vi "Icai 105v2.vi"() -> ()   [LabVIEW 2022 SP3]
uses:
  <vilib>/Utility/error.llb/DialogType.ctl
  <vilib>/DAQmx/write.llb/DAQmx Write (Analog DBL 1Chan 1Samp).vi
  <vilib>/DAQmx/write.llb/DAQmx Write (Analog Wfm 1Chan NSamp).vi
  <vilib>/DAQmx/create/channels.llb/DAQmx Create Channel (AO-Voltage-Basic).vi
  <vilib>/DAQmx/miscellaneous.llb/DAQmx Fill In Error Info.vi
  <vilib>/Waveform/WDTOps.llb/WDT Append Waveforms DBL.vi
  <vilib>/measure/NI_MABase.lvlib
panel:
  out "task out 2":refnum<k21> caption="task out"
  out "error out 2":errorcluster caption="error out (DAQ)"
  in  "Fs":dbl=1000000.0
  in  "?":T1(ring)=enum."Triangle Wave"
  in  "amplitude":dbl=1.0 format="%0.2p"
  in  "flat/ramp":bool
  in  "Ampl-RF \nend":dbl
  in  "Ampl-MW end":dbl=-1.0
  in  "Ampl-MW entry":dbl=-1.0
  in  "Ampl-RF \nentry":dbl
  in  "Ampl-RF T \npeak":dbl=5.0
  in  "Ampl-RF F\nborder peak":dbl=3.0
  in  "Amp-RF F\ncenter peak":dbl
  in  "RF gate":tag="Dev1/ao0"
  in  "FM Waveform Channel":tag="Dev1/ao2"
  out "task out":refnum<k21>
  out "error out":errorcluster caption="error out (DAQ)"
  out "Mod":dbl=118572.0
  out "Time-MW":dbl=3900000.0 format="%#_7g"
  out "Time-RF":dbl=3900000.0 format="%#_7g"
  in  "CAI/ICAI":bool=TRUE
  in  "DC 2":ext=1140.74 format="%.2f"
  out "Time- MW entry":dbl=579698.7113293351 format="%#_6f"
  in  "Fs":dbl=1000000.0
  out "#s":dbl=39524.02451426849
  in  "Time int":i32=7200
  in  "Sensitivity":u16(ring)=21 items=["2 nV/fA", "5 nV/fA", "10 nV/fA", "20 nV/fA", "50 nV/fA", "100 nV/fA", "200 nV/fA", "500 nV/fA", "1 uV/pA", "2 uV/pA", "5 uV/pA", "10 uV/pA", "20 uV/pA", "50 uV/pA", "100 uV/pA", "200 uV/pA", "500 uV/pA", "1 mV/nA", "2 mV/nA", "5 mV/nA", "10 mV/nA", "20 mV/nA", "50 mV/nA", "100 mV/nA", "200 mV/nA", "500 mV/nA", "1 V/uA"]
  in  "Detection Bandwidth":u16(ring)=7 items=["25 kHz", "8.33 kHz", "2.50 kHz", "833 Hz", "250 Hz", "83.3 Hz", "25 Hz", "8.33 Hz", "2.50 Hz", "0.833 Hz", "0.250 Hz", "0.0833 Hz", "0.025 Hz"]
  in  "SR 830 GPIB Address":i32=8
  in  "Freq 2":dbl=2290.0 format="%_7g"
  out "Iteration #":dbl=10.0
  in  "Iterations":dbl=2.0
  in  "stop 2":bool
  in  "pulse":bool=TRUE
  in  "Start":ext=0.2
  out "?":waveform(dbl)[](graph)=[{"t0"=timestamp(0 s since 1904-01-01), "dt"=1e-06, "Y"=array[3900000 elements]}, {"t0"=timestamp(0 s since 1904-01-01), "dt"=1e-06, "Y"=array[3900000 elements]}]
  in  "amplitude 2":dbl=1.0 format="%0.2p"
  in  "?":T1(ring)=enum."Triangle Wave"
  in  "phase 2":dbl format="%.2p"
  in  "Offset 2":dbl=-0.0 format="%#_6p"
  in  "frequency 4":dbl=100.0 format="%0.2p"
  in  "sampling info 4":cluster{"Fs":dbl, "#s":dbl}={"Fs"=1000000.0, "#s"=2500.0} {"Fs" format="%.2p"}
  in  "?":T1(ring)=enum."Triangle Wave"
  in  "offset 4":dbl=-1.0 format="%0.2p"
  in  "phase 4":dbl=90.0 format="%.2p"
  in  "amplitude 4":dbl=1.0 format="%0.2p"
  in  "frequency 1":dbl=100.0 format="%0.2p"
  in  "amplitude 1":dbl=1.0 format="%0.2p"
  in  "sampling info 1":cluster{"Fs":dbl, "#s":dbl}={"Fs"=1000000.0, "#s"=2500.0} {"Fs" format="%.2p"}
  in  "?":T1(ring)=enum."Triangle Wave"
  in  "phase 1":dbl=-90.0 format="%.2p"
  in  "Offset 1":dbl format="%#_6p"
  in  "iterat":dbl
  out "Time-MW osc":dbl=123571.0
  # "Iterat\ndetermines N times for For Loop on \n2 Traingle Wave's waveform (total length\nof waveform will be N+1)"
  # "DEFAULTS:"
  # "0"
  # "0"
  # "0"
  # "5"
  # "5"
  # "Mod\nDisplays the number of data points in\ntraingle wave 2's waveform after passing\nthrough a For Loop that adds itself to its\nend N times."
  # "DEFAULTS:"
  # "-1"
  # "-1"
  # "CW\nlength of the red form oscilating"
  # "controls the rf gate, the FM, & the AM"
  # "Ao Labeling\nInternal           external          function\nAo0                  Ao2                RF gate\nAo1                  Ao3                switch\nAo2                  Ao0                 FM\nAo3                   Ao1                AM"
  # "CAI/ICAI\nclose or not close the rf gate\nfor half of a period at the \nmiddle of the modulated wave\n(dark green)"
  # "Modulation Pulse"
  # "Pulse\nselects if the generated signal is\ngoing to be sent (bright green), or\nif only the results are shown in the\ngraph (dark green)"
  # "2"
  # "1"
  # "3"
  # "1 Triangle Wave\nbringing Beff to the x'-y' plane"
  # "2 Triangle Wave\ncoupling nuclear moment with\nthe cantilever at rf"
  # "3 Triangle Wave\nreturns the magnetization\nto the z axis"
  # "Detection Bandwith/ Sensitivity\nset the acquisition paramaters of\nthe lock-in amplifier during the\nmeasurements"
  # "DC 2\nsynchornize the phase of the\nmodulated wave with lock-in"
  # "Iteration\n# of times the continuus wave\nwill be applied"
  # "Start\nsets time delay between the rf gate\n& the beginning of the \noscillation of the modulation"
  # "rf gate trigger measures the length \nof the pulse and extends it, on both \nsides, by a quantity indicated in the start box"
  # "Mod\nSize of Y of waveform for\n2 Traingle Wave after passing \nthrough For Loop"
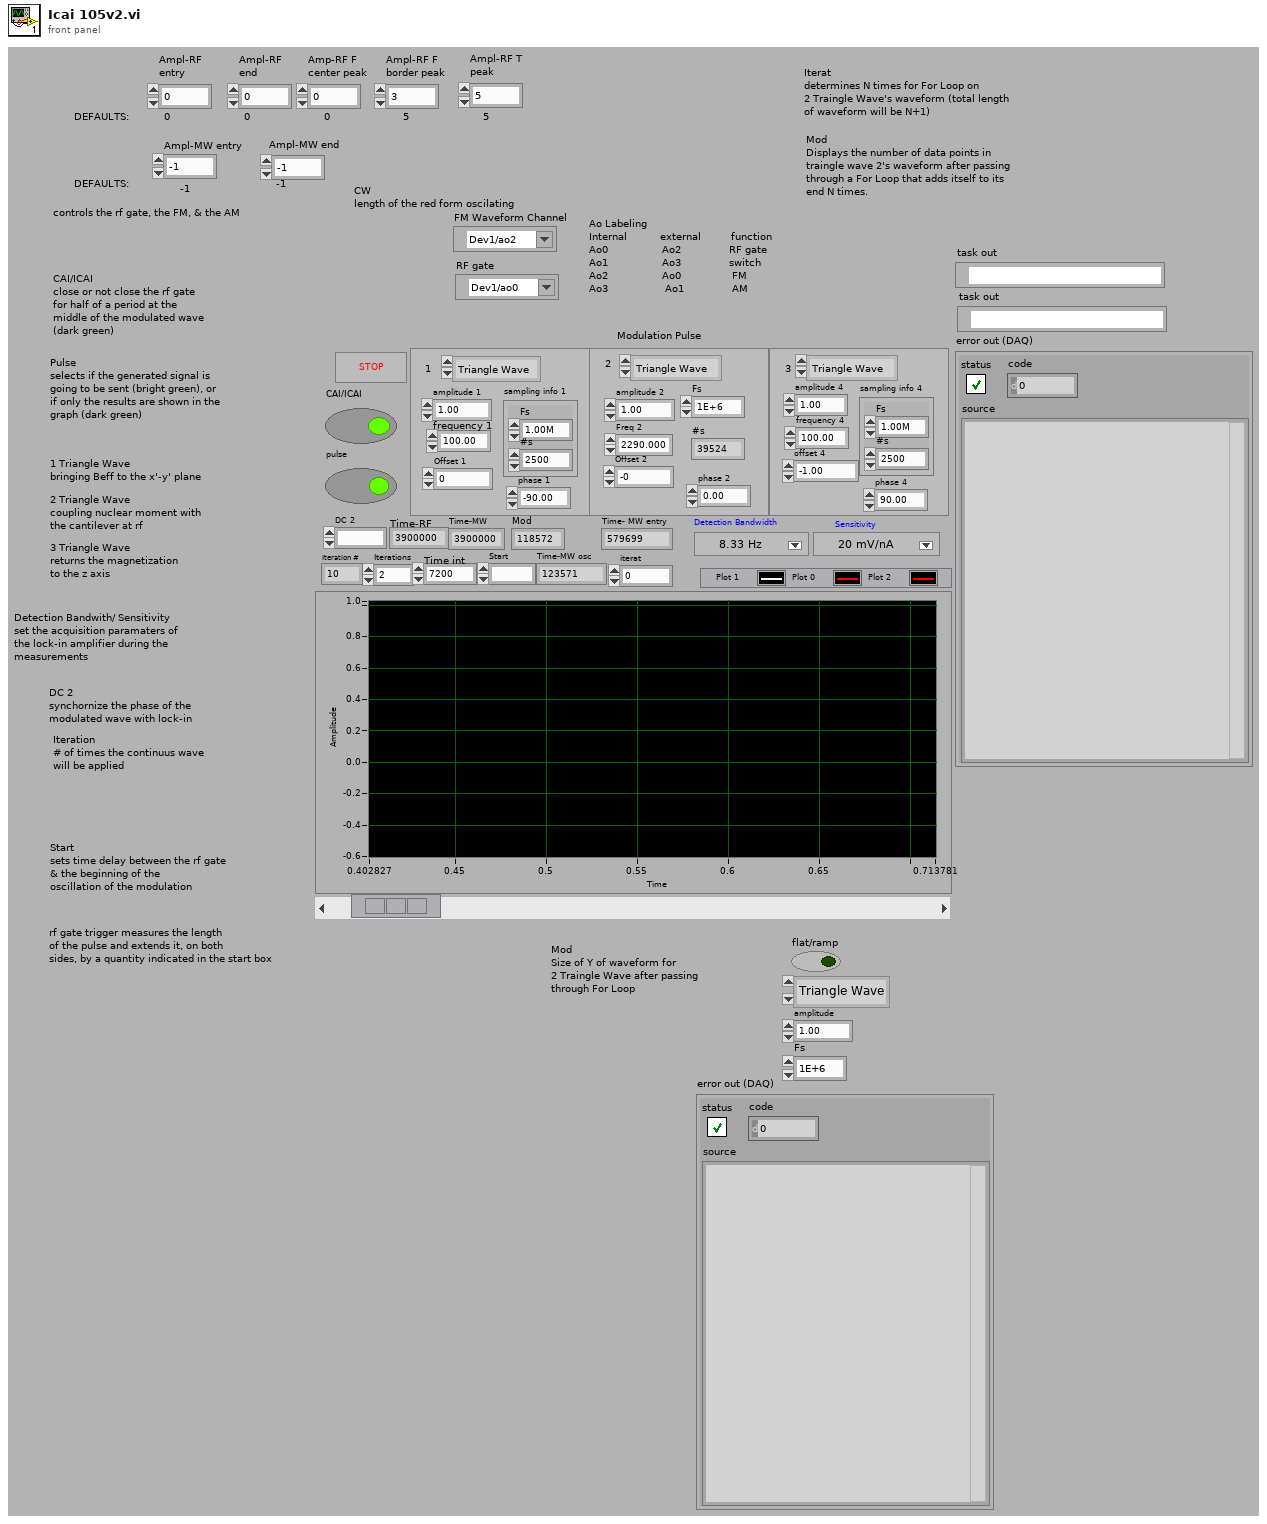
[diagram p1: front panel]
types:
  T1 = enum16{"Sine Wave", "Triangle Wave", "Square Wave", "Sawtooth Wave"}
  T2 = typedef "DialogType.ctl" = u16
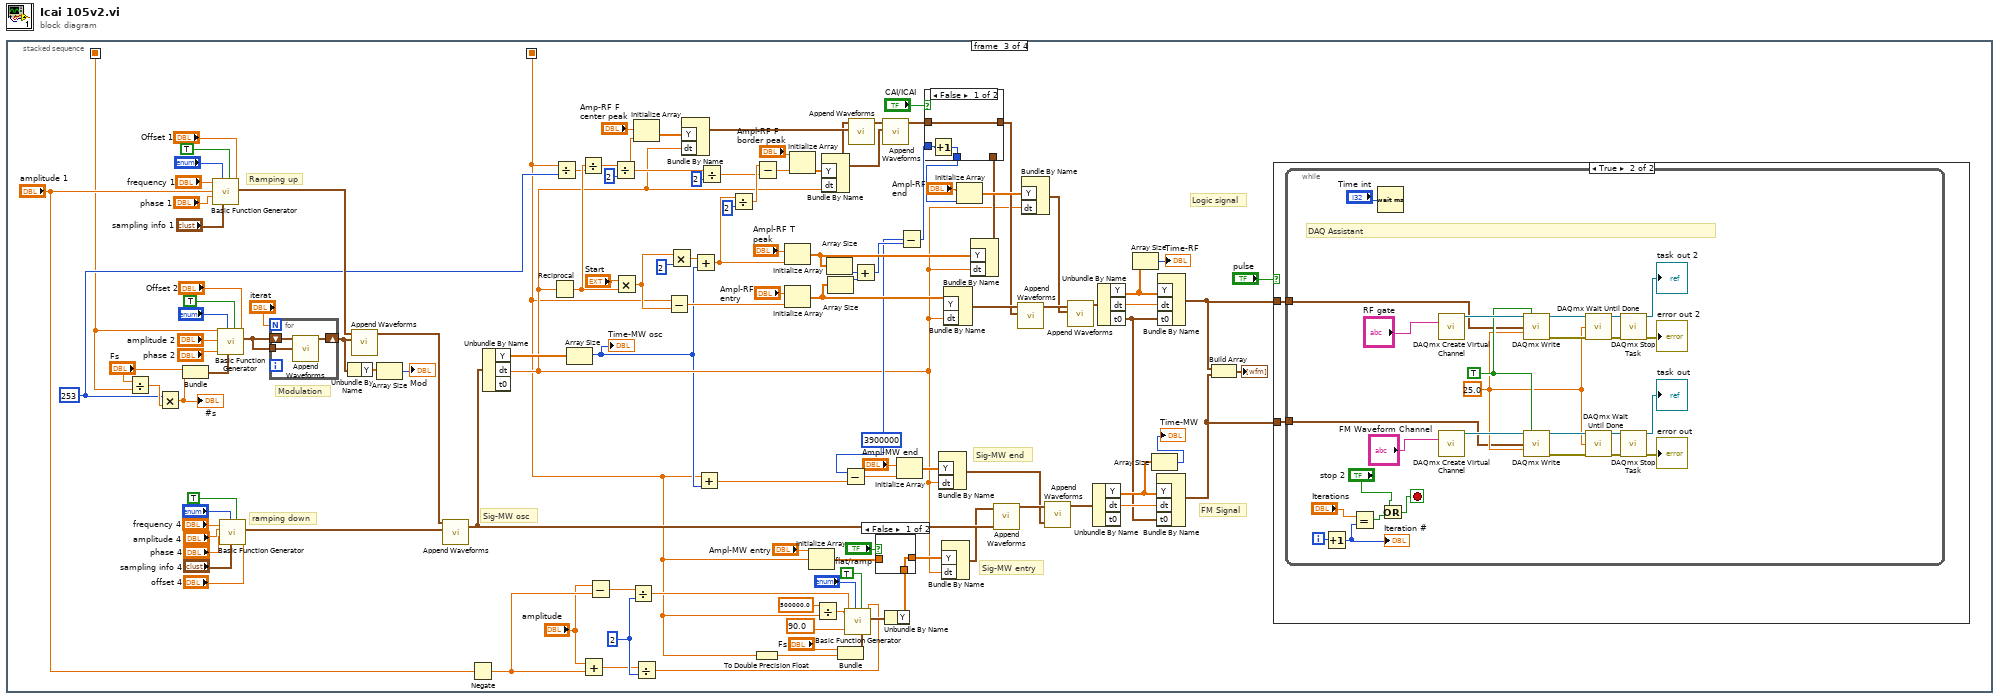
[diagram p0: block diagram]
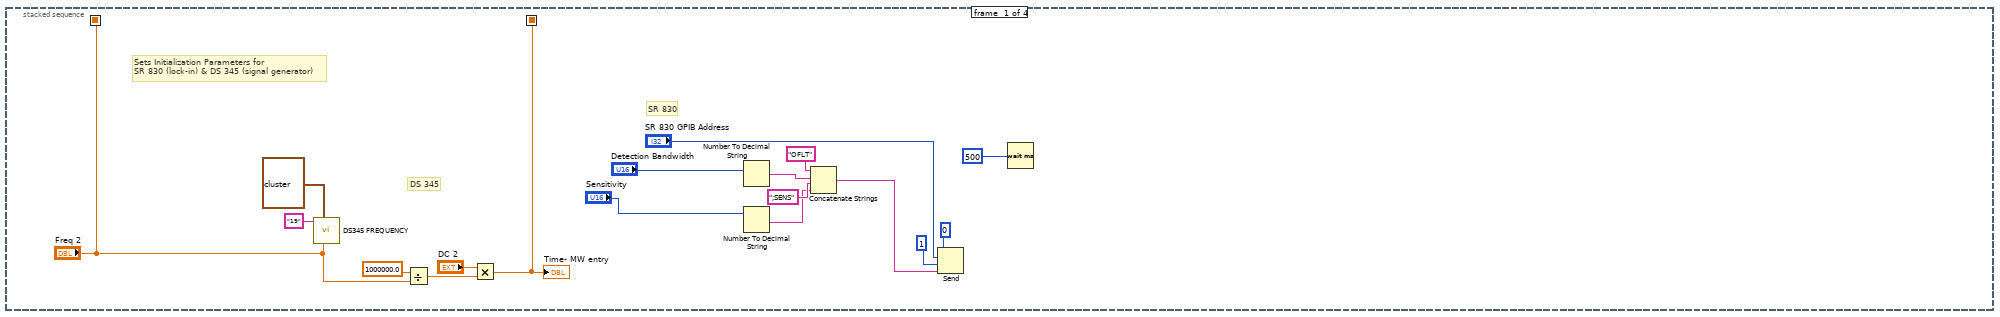
[diagram p2: hidden frame]
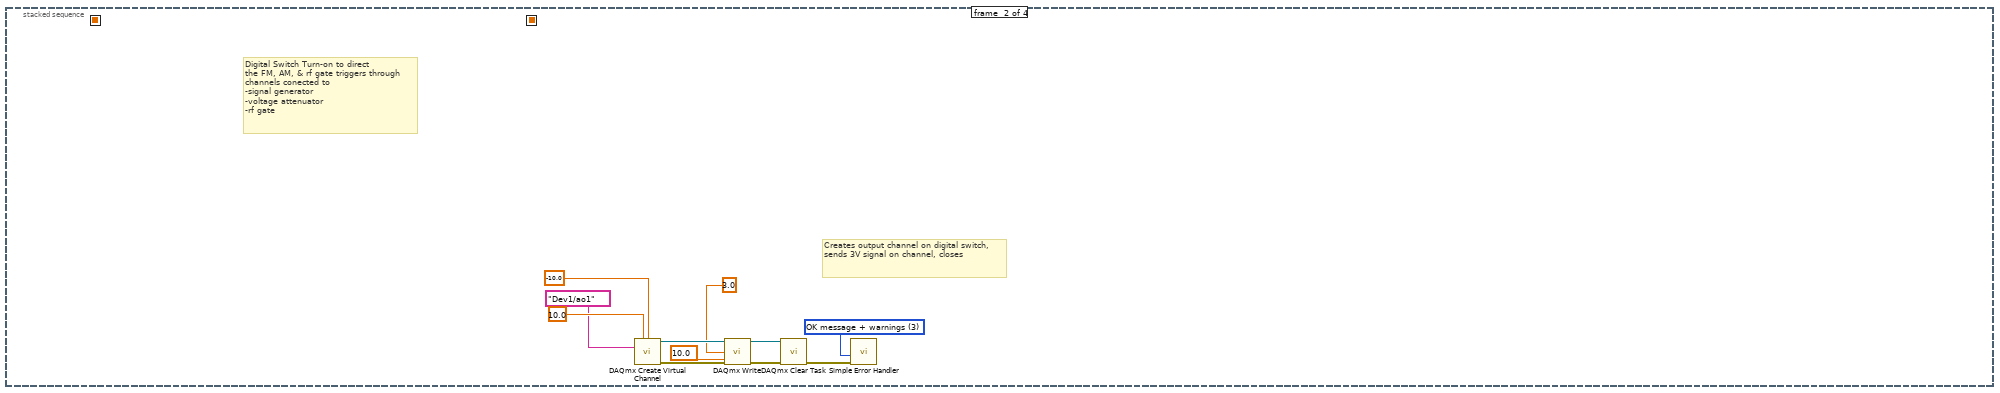
[diagram p3: hidden frame]
diagram:
  n1 = stacked-sequence {
    seq-local: ["Freq 2" _ _ _] -> [_ _ w30 _]
    seq-local: [w3 _ _ _] -> [_ _ w35 _]
    frame #0 {
      # "SR 830"
      # "DS 345"
      # "Sets Initialization Parameters for\nSR 830 (lock-in) & DS 345 (signal generator)"
      n2 = call "DS345 FREQUENCY.vi"("GPIB address"="19", "amplitude (0 Vrms:0)"=cluster{ext, i32} {0.02, 0} ("Driving amplitude (0 Vrms:0)"), "frequency"="Freq 2") -> ()  [unwired: 5 in, 1 out]
      n3 = Divide(x=1000000.0 ("Fs 2"), y="Freq 2") -> (x/y=w6:dbl)
      n4 = Multiply(x="DC 2", y=w6) -> (x*y=w3:ext)
      "Time- MW entry" <- w3
      n5 = Number To Decimal String(number="Detection Bandwidth") -> (decimal integer string=w15:string)  [unwired: 1 out]
      n6 = Number To Decimal String(number="Sensitivity") -> (decimal integer string=w13:string)  [unwired: 1 out]
      n7 = Concatenate Strings("OFLT", w15, ";SENS", w13) -> (w1:string)
      n8 = Send(0:0 ("bus"), 2:"SR 830 GPIB Address", 3:i16 1 ("mode"), 5:w1) -> ()  [unwired: 1 in, 3 out]
      n9 = Wait (ms)(milliseconds to wait=500) -> ()  [unwired: 1 out]
    }
    frame #1 {
      w22 = T2 3 items=["no dialog", "OK message", "continue or stop message", "OK message + warnings", "continue/stop + warnings"] ("type of dialog (OK msg:1)")
      # "Creates output channel on digital switch,\nsends 3V signal on channel, closes"
      # "Digital Switch Turn-on to direct\nthe FM, AM, & rf gate triggers through\nchannels conected to\n-signal generator\n-voltage attenuator\n-rf gate"
      n10 = call-poly <vilib>:"DAQmx Create Virtual Channel.vi"("maximum value"=10.0 ("Maximum Value"), "minimum value"=-10.0 ("Minimum Value"), "physical channels"=tag "Dev1/ao1" ("Physical Channel")) -> ("task out"=w25:refnum<k21>, "error out"=w26:errorcluster)  [unwired: 6 in, 5 out]
      n11 = call-poly <vilib>:"DAQmx Write.vi"("task/channels in"=w25, "data"=3.0 ("Voltage Output"), "timeout"=10.0, "error in"=w26) -> ("task out"=w20:refnum<k21>, "error out"=w21:errorcluster)  [unwired: 1 in, 9 out]
      n12 = call <vilib>:"DAQmx Clear Task.vi"("task in"=w20, "error in"=w21) -> ("error out"=w19:errorcluster)  [unwired: 13 out]
      n13 = call <vilib>:"Simple Error Handler.vi"("type of dialog (OK msg:1)"=w22, "error in (no error)"=w19) -> ()  [unwired: 8 out]
    }
    frame #2 {
      w50 = 2
      w88 = 253
      w40 = 3900000
      # "Sig-MW end"
      # "Sig-MW entry"
      # "Sig-MW osc"
      # "FM Signal"
      # "Logic signal"
      # "Ramping up"
      # "ramping down"
      # "Modulation"
      n14 = Divide(x="Fs", y=w30) -> (x/y=w107:dbl)
      n15 = Multiply(x=w88, y=w107) -> (x*y=w105:dbl)
      "#s" <- w105
      n16 = Bundle("Fs"="Fs", w105) -> (w104:cluster{"Fs":dbl, dbl})  [unwired: 1 out]
      n17 = call <vilib>:"Basic Function Generator.vi"("offset"="Offset 1", "reset signal"=TRUE, "sampling info"="sampling info 1", "signal type"="?", "phase"="phase 1", "amplitude"="amplitude 1", "frequency"="frequency 1") -> ("signal out"=w132:waveform(dbl))  [unwired: 2 in, 2 out]
      n18 = call <vilib>:"Basic Function Generator.vi"("offset"="Offset 2", "reset signal"=TRUE, "sampling info"=w104, "signal type"="?", "phase"="phase 2", "amplitude"="amplitude 2", "frequency"=w30) -> ("signal out"=w108:waveform(dbl))  [unwired: 2 in, 2 out]
      n19 = call <vilib>:"Basic Function Generator.vi"("offset"="offset 4", "reset signal"=TRUE, "sampling info"="sampling info 4", "signal type"="?", "phase"="phase 4", "amplitude"="amplitude 4", "frequency"="frequency 4") -> ("signal out"=w136:waveform(dbl))  [unwired: 2 in, 2 out]
      n20 = for {
        N: "iterat" -> [_]
        shift-right: [w189] -> w77
        shift-left: w108 -> [w187]
        tunnel: w108 -> [w188]
        n21 = call-poly <vilib>:"Append Waveforms.vi"("waveform B"=w188, "waveform A"=w187) -> ("waveform out"=w189:waveform(dbl))  [unwired: 1 in, 8 out]
      }
      n22 = Unbundle By Name(w77) -> ("Y"=w78:dbl[])
      n23 = call-poly <vilib>:"Append Waveforms.vi"("waveform B"=w77, "waveform A"=w132) -> ("waveform out"=w131:waveform(dbl))  [unwired: 1 in, 8 out]
      n24 = Array Size(array=w78) -> (size(s)=→"Mod":i32)
      n25 = call-poly <vilib>:"Append Waveforms.vi"("waveform B"=w136, "waveform A"=w131) -> ("waveform out"=w130:waveform(dbl))  [unwired: 1 in, 8 out]
      n26 = Negate(x="amplitude 1") -> (-x=w48:dbl)
      n27 = Unbundle By Name ("Get Waveform Components")(w130) -> ("Y"=w133:dbl[], "dt"=w37:dbl)  [unwired: 1 out]
      n28 = Reciprocal(x=w37) -> (1/x=w97:dbl)
      n29 = Divide(x=w35, y=w88) -> (x/y=w96:ext)
      n30 = Array Size(array=w133) -> (size(s)=w36:i32)
      "Time-MW osc" <- w36
      n31 = Divide(x=w97, y=w96) -> (x/y=w94:ext)
      n32 = Add(x="amplitude", y=w48) -> (x+y=w41:dbl)
      n33 = Subtract(x="amplitude", y=w48) -> (x-y=w49:dbl)
      n34 = Divide(x=w94, y=2) -> (x/y=w91:ext)
      n35 = Multiply(x="Start", y=w97) -> (x*y=w115:ext)
      n36 = Divide(x=w49, y=w50) -> (x/y=w45:dbl)
      n37 = Initialize Array("Amp-RF F\ncenter peak", w91) -> (w100:dbl[])
      n38 = Divide(x=w41, y=w50) -> (x/y=w46:dbl)
      n39 = Subtract(x=w35, y=w115) -> (x-y=w116:ext)
      n40 = Multiply(x=w115, y=2) -> (x*y=w120:ext)
      n41 = Bundle By Name("Y"=w100, "dt"=w37) -> (w99:waveform(dbl))  [unwired: 1 out]
      n42 = Add(x=w120, y=w36) -> (x+y=w103:ext)
      n43 = Add(x=w35, y=w36) -> (x+y=w122:ext)
      n44 = Divide(x=w91, y=2) -> (x/y=w89:ext)
      n45 = Divide(x=w103, y=2) -> (x/y=w93:ext)
      n46 = To Double Precision Float(number=w35) -> (double precision float=w58:dbl)
      n47 = Subtract(x=w93, y=w89) -> (x-y=w92:ext)
      n48 = Initialize Array("Ampl-RF T \npeak", w103) -> (w114:dbl[])
      n49 = Initialize Array("Ampl-RF \nentry", w116) -> (w65:dbl[])
      n50 = Initialize Array("Ampl-RF F\nborder peak", w92) -> (w101:dbl[])
      n51 = Initialize Array("Ampl-MW entry", w35) -> (w57:dbl[])
      n52 = Divide(x=500000.0, y=w35) -> (x/y=w53:ext)
      n53 = Bundle By Name("Y"=w101, "dt"=w37) -> (w44:waveform(dbl))  [unwired: 1 out]
      n54 = Array Size(array=w114) -> (size(s)=w112:i32)
      n55 = Array Size(array=w65) -> (size(s)=w113:i32)
      n56 = Bundle("Fs"="Fs", w58) -> (w59:cluster{"Fs":dbl, dbl})  [unwired: 1 in]
      n57 = Subtract(x=w40, y=w122) -> (x-y=w52:ext)
      n58 = call <vilib>:"Basic Function Generator.vi"("offset"=w46, "reset signal"=TRUE, "sampling info"=w59, "signal type"="?", "phase"=90.0 ("phase 3"), "amplitude"=w45, "frequency"=w53) -> ("signal out"=w62:waveform(dbl))  [unwired: 2 in, 2 out]
      n59 = call-poly <vilib>:"Append Waveforms.vi"("waveform B"=w99, "waveform A"=w44) -> ("waveform out"=w98:waveform(dbl))  [unwired: 1 in, 8 out]
      n60 = Add(x=w112, y=w113) -> (x+y=w111:i32)
      n61 = call-poly <vilib>:"Append Waveforms.vi"("waveform B"=w44, "waveform A"=w98) -> ("waveform out"=w87:waveform(dbl))  [unwired: 1 in, 8 out]
      n62 = Unbundle By Name(w62) -> ("Y"=w56:dbl[])
      n63 = case shown="False" "flat/ramp" {
        tunnel: w57 -> [_ w152]
        tunnel: w56 -> [w151 _]
        tunnel: [w151 w152] -> w55
        frame False {
        }
        frame True {
        }
      }
      n64 = Initialize Array("Ampl-MW end", w52) -> (w121:dbl[])
      n65 = Subtract(x=w40, y=w111) -> (x-y=w68:i32)
      n66 = Bundle By Name("Y"=w121, "dt"=w37) -> (w32:waveform(dbl))  [unwired: 1 out]
      n67 = Bundle By Name("Y"=w55, "dt"=w37) -> (w34:waveform(dbl))  [unwired: 1 out]
      n68 = Bundle By Name("Y"=w65, "dt"=w37) -> (w118:waveform(dbl))  [unwired: 1 out]
      n69 = Bundle By Name("Y"=w114, "dt"=w37) -> (w85:waveform(dbl))  [unwired: 1 out]
      n70 = case shown="False" "CAI/ICAI" {
        tunnel: w87 -> [w155 _]
        tunnel: [w155 w157] -> w86
        tunnel: w85 -> [_ w157]
        tunnel: w68 -> [w154 w156]
        tunnel: [w153 w156] -> w67
        frame False {
          n71 = Increment(x=w154) -> (x+1=w153:i32)
        }
        frame True {
        }
      }
      n72 = Initialize Array("Ampl-RF \nend", w67) -> (w119:dbl[])
      n73 = call-poly <vilib>:"Append Waveforms.vi"("waveform B"=w130, "waveform A"=w34) -> ("waveform out"=w135:waveform(dbl))  [unwired: 1 in, 8 out]
      n74 = call-poly <vilib>:"Append Waveforms.vi"("waveform B"=w86, "waveform A"=w118) -> ("waveform out"=w129:waveform(dbl))  [unwired: 1 in, 8 out]
      n75 = Bundle By Name("Y"=w119, "dt"=w37) -> (w117:waveform(dbl))  [unwired: 1 out]
      n76 = call-poly <vilib>:"Append Waveforms.vi"("waveform B"=w32, "waveform A"=w135) -> ("waveform out"=w125:waveform(dbl))  [unwired: 1 in, 8 out]
      n77 = call-poly <vilib>:"Append Waveforms.vi"("waveform B"=w117, "waveform A"=w129) -> ("waveform out"=w127:waveform(dbl))  [unwired: 1 in, 8 out]
      n78 = Unbundle By Name(w125) -> ("Y"=w80:dbl[], "dt"=w124:dbl)  [unwired: 1 out]
      n79 = Unbundle By Name(w127) -> ("Y"=w82:dbl[], "dt"=w126:dbl, "t0"=w33:timestamp)
      n80 = Array Size(array=w82) -> (size(s)=→"Time-RF":i32)
      n81 = Array Size(array=w80) -> (size(s)=→"Time-MW":i32)
      n82 = Bundle By Name("Y"=w80, "dt"=w124, "t0"=w33) -> (w39:waveform(dbl))  [unwired: 1 out]
      n83 = Bundle By Name("Y"=w82, "dt"=w126, "t0"=w33) -> (w38:waveform(dbl))  [unwired: 1 out]
      n84 = Build Array(w38, w39) -> (→"?":waveform(dbl)[])
      n85 = case shown="True" "pulse" {
        tunnel: w38 -> [_ w159]
        tunnel: w39 -> [_ w158]
        frame False {
        }
        frame True {
          n86 = while {
            tunnel: w159 -> [w162]
            tunnel: w158 -> [w163]
            i -> [w183]
            stop <- w184 stop-if-true
            w165 = TRUE ("auto start")
            w164 = 25.0 ("timeout (s)")
            # "DAQ Assistant"
            n87 = Increment(x=w183) -> (x+1=w181:i32)
            "Iteration #" <- w181
            n88 = Equal?(x="Iterations", y=w181) -> (x = y?=w186:bool)
            n89 = Wait (ms)(milliseconds to wait="Time int") -> ()  [unwired: 1 out]
            n90 = Or(x="stop 2", y=w186) -> (x .or. y?=w184:bool)
            n91 = call-poly <vilib>:"DAQmx Create Virtual Channel.vi"("physical channels"="RF gate") -> ("task out"=w172:refnum<k21>)  [unwired: 13 in, 1 out]
            n92 = call-poly <vilib>:"DAQmx Create Virtual Channel.vi"("physical channels"="FM Waveform Channel") -> ("task out"=w173:refnum<k21>)  [unwired: 13 in, 1 out]
            n93 = call-poly <vilib>:"DAQmx Write.vi"("task/channels in"=w172, "auto start"=w165, "data"=w162, "timeout"=w164) -> ("task out"=w171:refnum<k21>, "error out"=w166:errorcluster)  [unwired: 9 in, 1 out]
            n94 = call-poly <vilib>:"DAQmx Write.vi"("task/channels in"=w173, "auto start"=w165, "data"=w163, "timeout"=w164) -> ("task out"=w175:refnum<k21>, "error out"=w174:errorcluster)  [unwired: 9 in, 1 out]
            n95 = call <vilib>:"DAQmx Wait Until Done.vi"("task/channels in"=w171, "timeout (sec)"=w164, "error in"=w166) -> ("task out"=w170:refnum<k21>, "error out"=w167:errorcluster)  [unwired: 11 in]
            n96 = call <vilib>:"DAQmx Wait Until Done.vi"("task/channels in"=w175, "timeout (sec)"=w164, "error in"=w174) -> ("task out"=w179:refnum<k21>, "error out"=w178:errorcluster)  [unwired: 11 in]
            n97 = call <vilib>:"DAQmx Stop Task.vi"("task/channels in"=w170, "error in"=w167) -> ("task out"=→"task out 2":refnum<k21>, "error out"=→"error out 2":errorcluster)  [unwired: 12 in]
            n98 = call <vilib>:"DAQmx Stop Task.vi"("task/channels in"=w179, "error in"=w178) -> ("task out"=→"task out":refnum<k21>, "error out"=→"error out":errorcluster)  [unwired: 12 in]
          }
        }
      }
    }
    frame #3 {
    }
  }
